vi "TcpCilent.vi"() -> ()   [LabVIEW 2021]
doc: "Demonstrates how to open a connection to an TCP server, read the data being sent, and display the data on a chart. This VI is designed to stop if the TCP connection is terminated."
panel:
  out "?":dbl format="%%%.1f"
  out "progress":dbl(slide) scale=0.0..100.0
  in  "?":path
  in  "Server Closed":string="The server VI closed the connection."
  # "click here to choose where\nto store files"
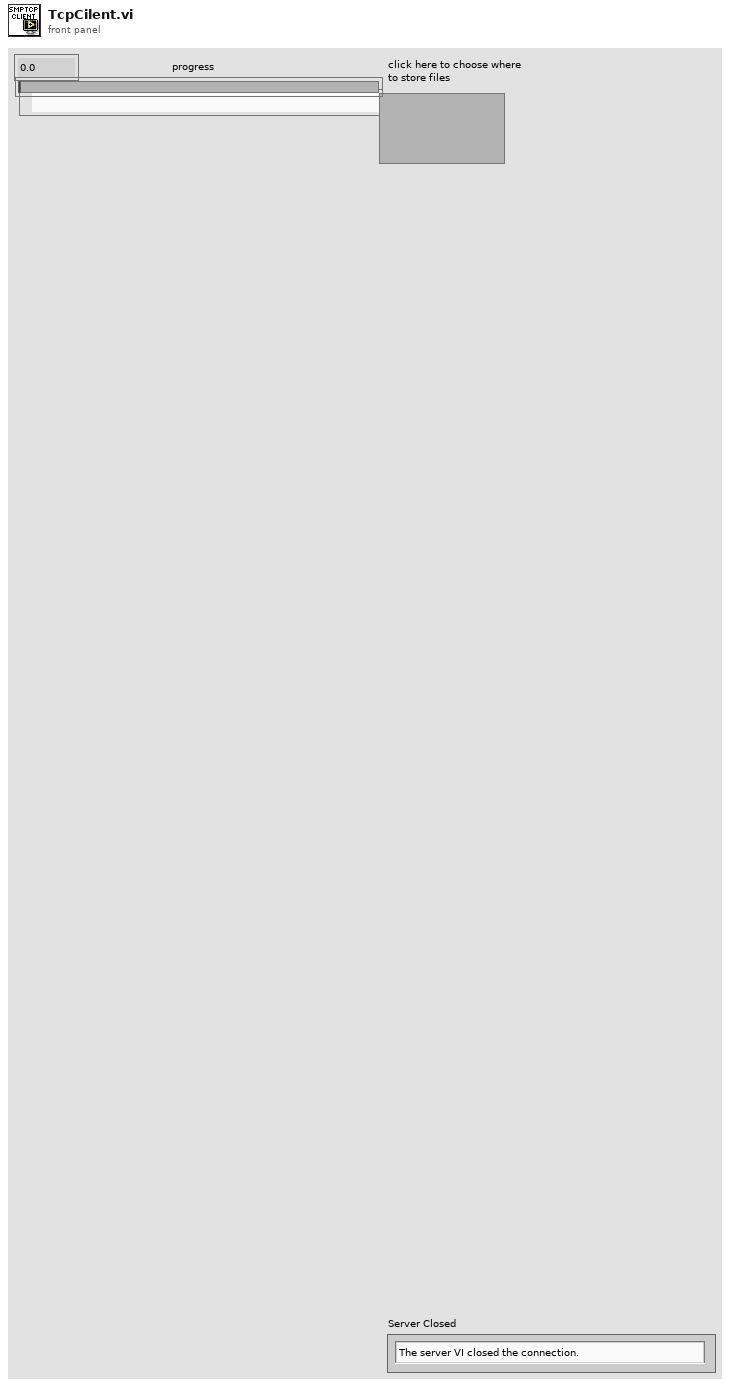
[diagram p1: front panel]
types:
  T1 = enum16{"open", "replace", "create", "open or create", "replace or create", "replace or create with confirmation"}
  T2 = enum16{"big-endian, network order", "native, host order", "little-endian"}
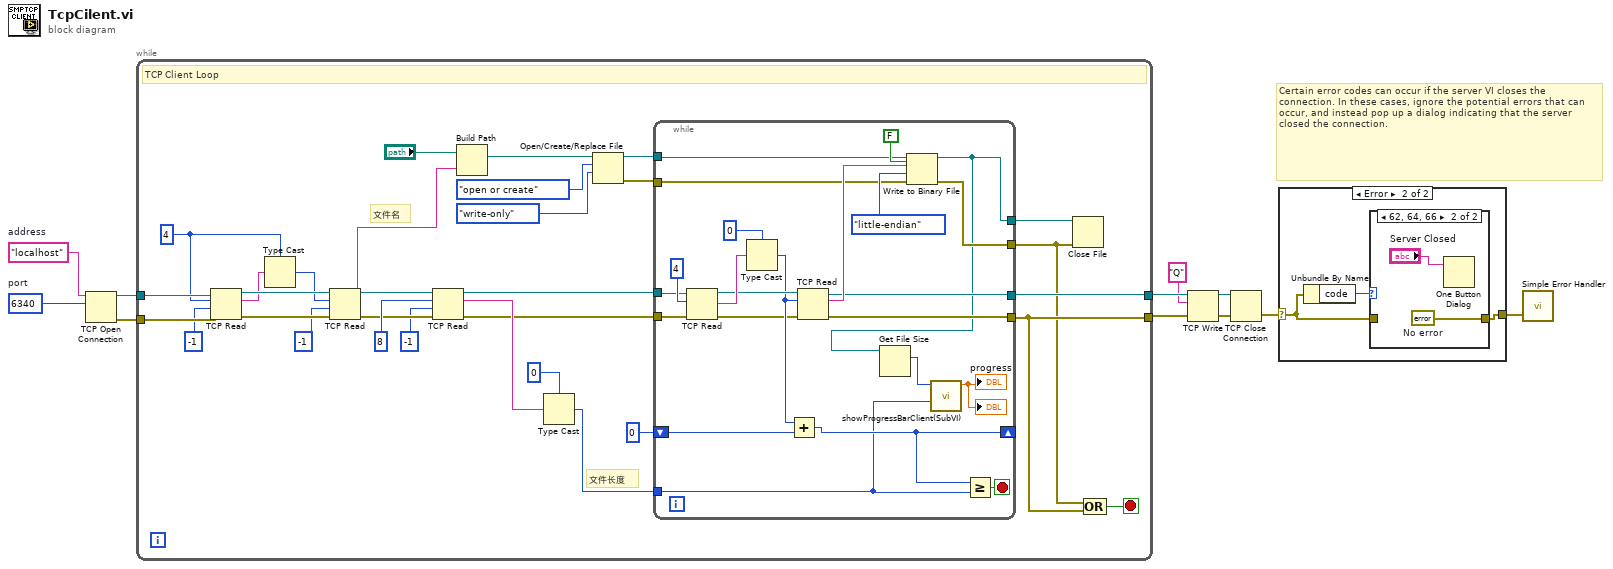
[diagram p0: block diagram]
diagram:
  w2 = u16 6340  # port
  w3 = "localhost"  # address
  # "Certain error codes can occur if the server VI closes the connection. In these cases, ignore the potential errors that can occur, and instead pop up a dialog indicating that the server closed the connection."
  n1 = TCP Open Connection(address=w3, remote port or service name=w2) -> (connection ID=w11:refnum<k5>, error out=w10:errorcluster)  [unwired: 3 in]
  n2 = while {
    tunnel: w10 -> [w40]
    tunnel: w11 -> [w42]
    tunnel: [w17] -> w8
    tunnel: [w15] -> w1
    stop <- w13 stop-if-true
    w37 = 4 ("bytes to read")
    # "文件长度"
    # "文件名"
    # "TCP Client Loop"
    n3 = TCP Read(connection ID=w42, bytes to read=w37, error in (no error)=w40, 9:-1 ("timeout ms (25000)")) -> (connection ID out=w41:refnum<k5>, data out=w38:string, error out=w39:errorcluster)  [unwired: 1 in]
    n4 = Type Cast(type=w37, x=w38) -> (*(type *) &x=w36:i32)
    n5 = TCP Read(connection ID=w41, bytes to read=w36, error in (no error)=w39, 9:-1 ("timeout ms (25000)")) -> (connection ID out=w23:refnum<k5>, data out=w33:string, error out=w22:errorcluster)  [unwired: 1 in]
    n6 = TCP Read(connection ID=w23, bytes to read=8, error in (no error)=w22, 9:-1 ("timeout ms (25000)")) -> (connection ID out=w25:refnum<k5>, data out=w24:string, error out=w16:errorcluster)  [unwired: 1 in]
    n7 = Build Path(base path="?", name or relative path=w33) -> (appended path=w32:path)
    n8 = Type Cast(type=i64 0, x=w24) -> (*(type *) &x=w29:i64)
    n9 = Open/Create/Replace File(file path (use dialog)=w32, operation (0:open)=T1."open or create", access (0:read/write)=enum16{"read/write", "read-only", "write-only"}."write-only") -> (refnum out=w12:refnum<file>, error out=w18:errorcluster)  [unwired: 3 in, 1 out]
    n10 = while {
      tunnel: w29 -> [w47]
      shift-right: [w48] -> _
      shift-left: 0 -> [w65]
      tunnel: w25 -> [w63]
      tunnel: w12 -> [w45]
      tunnel: [w44] -> w26
      tunnel: [w54] -> w14
      tunnel: w18 -> [w53]
      tunnel: [w52] -> w17
      tunnel: w16 -> [w50]
      tunnel: [w49] -> w15
      stop <- w58 stop-if-true
      n11 = TCP Read(connection ID=w63, bytes to read=4, error in (no error)=w50) -> (connection ID out=w60:refnum<k5>, data out=w62:string, error out=w51:errorcluster)  [unwired: 2 in]
      n12 = Type Cast(type=0, x=w62) -> (*(type *) &x=w59:i32)
      n13 = Add(x=w59, y=w65) -> (x+y=w48:i32)
      n14 = TCP Read(connection ID=w60, bytes to read=w59, error in (no error)=w51) -> (connection ID out=w52:refnum<k5>, data out=w57:string, error out=w49:errorcluster)  [unwired: 2 in]
      n15 = Write to Binary File(file (use dialog)=w45, data=w57, error in=w53, 5:FALSE ("prepend array or string size? (T)"), 9:T2."little-endian" ("byte order (0:big-endian, network order)")) -> (refnum out=w44:refnum<file>, error out=w54:errorcluster)  [unwired: 1 in, 1 out]
      n16 = Get File Size(file=w44) -> (size (in bytes)=w46:i64)  [unwired: 1 in, 2 out]
      n17 = call "showProgressBarClient(SubVI).vi"("file size"=w47, "received"=w46) -> ("progress"=→"progress" →"?":dbl)  [unwired: 9 in]
      n18 = Greater Or Equal?(x=w48, y=w47) -> (x >= y?=w58:bool)
    }
    n19 = Close File(refnum=w26, error in=w14) -> ()  [unwired: 2 out]
    n20 = Compound Arithmetic op=OR(w14, w15) -> (w13:bool)
  }
  n21 = TCP Write(connection ID=w8, data in="Q", error in (no error)=w1) -> (connection ID out=w9:refnum<k5>, error out=w7:errorcluster)  [unwired: 2 out]
  n22 = TCP Close Connection(connection ID=w9, error in (no error)=w7) -> (error out=w5:errorcluster)  [unwired: 1 in, 1 out]
  n23 = case shown="Error" w5 {
    selector: w5 -> [w66 w68]
    tunnel: [w66 w67] -> w4
    frame No Error {
    }
    frame Error {
      n24 = Unbundle By Name(w68) -> ("code"=w69:i32)
      n25 = case shown="62, 64, 66" w69 {
        tunnel: w68 -> [w70 _]
        tunnel: [w70 w72] -> w67
        frame Default {
        }
        frame 62, 64, 66 {
          w72 = errorcluster {"status"=FALSE, "code"=0, "source"=""}  # No error
          n26 = One Button Dialog(message="Server Closed") -> ()  [unwired: 1 in, 1 out]
        }
      }
    }
  }
  n27 = call <vilib>:"Simple Error Handler.vi"("error in (no error)"=w4) -> ()  [unwired: 4 in, 5 out]
